vi "GetText.vi"(8 "error in":errorcluster, 11 "node in":refnum<class "VIPB Build Node.lvclass">) -> (0 "error out":errorcluster, 1 "additional text":string, 2 "text":string, 3 "node out":refnum<class "VIPB Build Node.lvclass">, 4 "glyph":string)   [LabVIEW 2014, in "VIPB Build Node.lvclass"]
doc: "Returns the text representation of the node used for the tree control.Copyright 2015 National Instruments Corporation\n\nLicensed under the Apache License, Version 2.0 (the \"License\"); you may not use this file except in compliance with the License. You may obtain a copy of the License at http://www.apache.org/licenses/LICENSE-2.0\nUnless required by applicable law or agreed to in writing, software distributed under the License is distributed on an \"AS IS\" BASIS, WITHOUT WARRANTIES OR CONDITIONS OF ANY KIND, either express or implied. See the License for the specific language governing permissions and limitations under the License."
uses:
  VIPB Build Node.lvclass
  VIPB Build Node.lvclass/VIPB Build Node.ctl
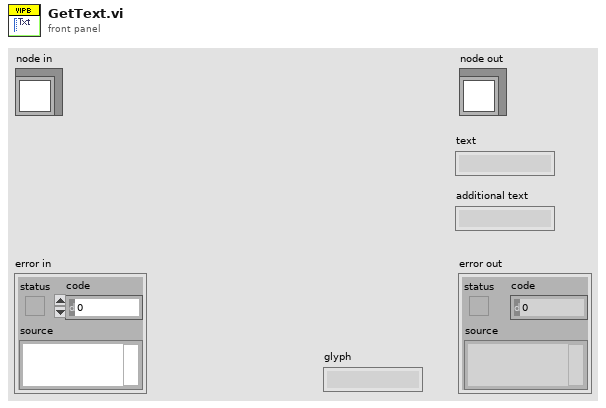
[diagram p1: front panel]
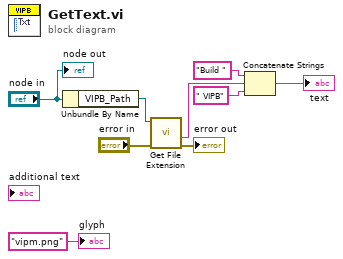
[diagram p0: block diagram]
diagram:
  n1 = Unbundle By Name("node in") -> ("VIPB_Path"=w6:path)
  n2 = call <vilib>:"Get File Extension.vi"("error in (no error)"="error in", "file"=w6) -> ("error out"=→"error out":errorcluster, "filename without extension"=w8:string)  [unwired: 6 in, 2 out]
  n3 = Concatenate Strings("Build " ("string"), w8, " VIPB" ("string")) -> (→"text":string)
  "node out" <- "node in"
  "glyph" <- "vipm.png" ("glyph")
